vi "generate 1 cycle.vi"(8 "error in (no error)":errorcluster caption="에러 입력(에러 없음)", 11 "Sawtooth Wave 입력":refnum<class "Sawtooth Wave.lvclass">) -> (0 "error out":errorcluster caption="에러 출력", 2 "waveform out":waveform(dbl), 3 "Sawtooth Wave 출력":refnum<class "Sawtooth Wave.lvclass">)   [LabVIEW 2020, in "Sawtooth Wave.lvclass"]
uses:
  Sawtooth Wave.lvclass
  Waveform Gen/Waveform Gen.lvclass/Waveform Gen.ctl
  Waveform Obj/Waveform Obj.lvclass/Waveform Obj.ctl
  Waveform Gen/Accessors/Read frequency.vi
  Waveform Gen/Accessors/Read scale.vi
  Waveform Gen/Accessors/Read phase.vi
  Waveform Obj/Accessors/Read sampling rate.vi
  <vilib>/measure/NI_MABase.lvlib
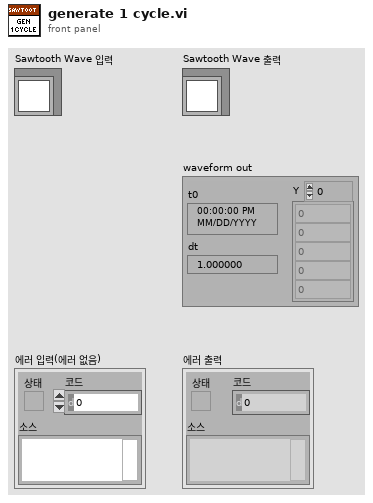
[diagram p1: front panel]
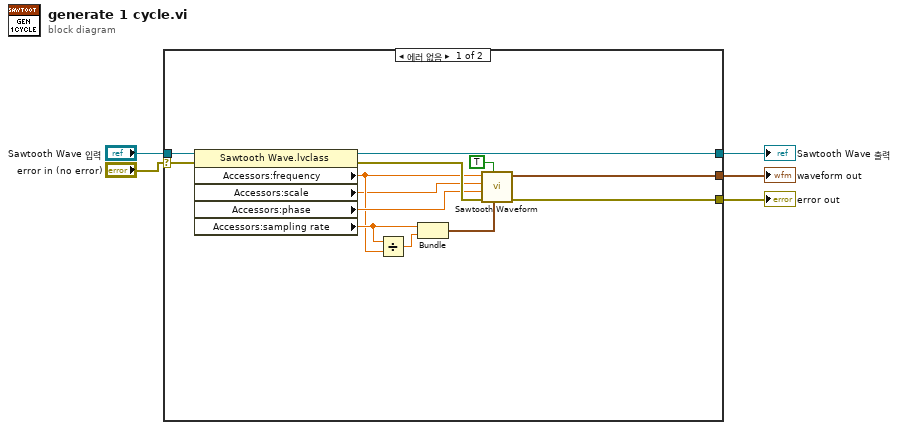
[diagram p0: block diagram]
diagram:
  n1 = case shown="에러 없음" "error in (no error)" {
    selector: "error in (no error)" -> [w10 w20]
    tunnel: [w7 w20] -> w2
    tunnel: "Sawtooth Wave 입력" -> [w17 w19]
    tunnel: [w8 w19] -> w4
    tunnel: [w6 _] -> w1
    frame No Error {
      n2 = property class="Sawtooth Wave.lvclass"(reference=w17, error in=w10) -> (reference out=w8:refnum<class "Sawtooth Wave.lvclass">, error out=w18:errorcluster, "Accessors:frequency"=w14:dbl, "Accessors:scale"=w9:dbl, "Accessors:phase"=w16:dbl, "Accessors:sampling rate"=w15:dbl)
      n3 = Divide(x=w15, y=w14) -> (x/y=w13:dbl)
      n4 = Bundle("Accessors:sampling rate"=w15, w13) -> (w12:cluster{"Accessors:sampling rate":dbl, dbl})  [unwired: 1 in]
      n5 = call <vilib>:"Sawtooth Waveform.vi"("sampling info"=w12, "reset signal"=TRUE, "error in (no error)"=w18, "phase"=w16, "amplitude"=w9, "frequency"=w14) -> ("error out"=w7:errorcluster, "signal out"=w6:waveform(dbl))  [unwired: 4 in]
    }
    frame Error {
    }
  }
  "error out" <- w2
  "Sawtooth Wave 출력" <- w4
  "waveform out" <- w1
